vi "YAFTAF_Create.vi"(8 "ErrorIn":errorcluster, 11 "ObjectIn":refnum<class "YAFTAF.lvclass">) -> (0 "ErrorOut":errorcluster, 3 "ObjectOut":refnum<class "YAFTAF.lvclass">)   [LabVIEW 2021, in "YAFTAF.lvclass"]
uses:
  YAFTAF.lvclass
  C:/Localdata/Projects/TriekselSoft/TriekselsoftApplicationFramework/Source/.Externals/Library_YAF/YActor/YActor.lvclass
  YAFTAF_Constructor.vi
  YAFTAF_UserInterface.vi
  YActor/YActor.lvclass
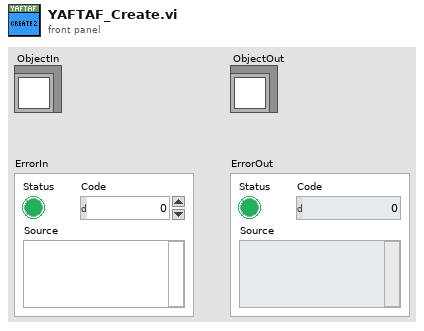
[diagram p1: front panel]
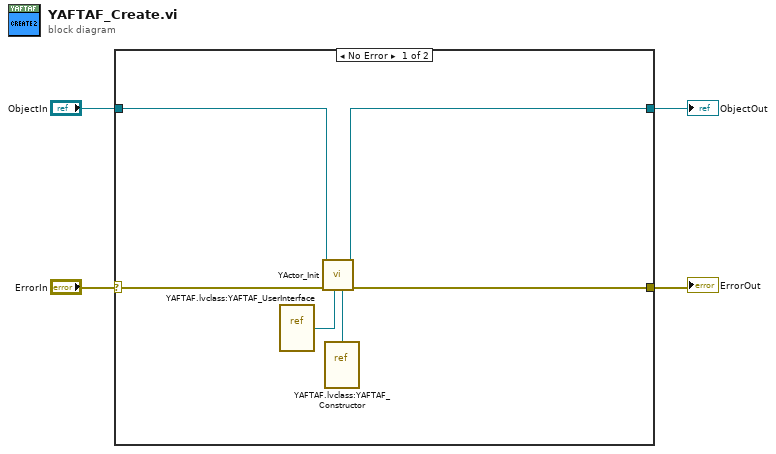
[diagram p0: block diagram]
diagram:
  n1 = case shown="No Error" "ErrorIn" {
    selector: "ErrorIn" -> [w9 w12]
    tunnel: [w10 w12] -> w3
    tunnel: [w6 w11] -> w1
    tunnel: "ObjectIn" -> [w5 w11]
    frame No Error {
      n2 = vi-ref "YAFTAF.lvclass:YAFTAF_UserInterface.vi"() -> (w7:refnum<vi>)
      n3 = vi-ref "YAFTAF.lvclass:YAFTAF_Constructor.vi"() -> (w8:refnum<vi>)
      n4 = call "YActor_Init.vi"("ConstructorRef"=w8, "ActorRef(EmptyRef=StandardActor)"=w7, "ErrorIn"=w9, "YActorIn"=w5) -> ("ErrorOut"=w10:errorcluster, "YActorOut"=w6:refnum<class "YAFTAF.lvclass">)  [unwired: 6 in]
    }
    frame Error {
    }
  }
  "ErrorOut" <- w3
  "ObjectOut" <- w1
